vi "AddSubVIInline.vi"(9 "Numeric 3":i32, 10 "Numeric in":i32) -> (2 "Numeric out":i32)   [LabVIEW 2016]
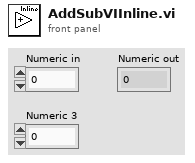
[diagram p1: front panel]
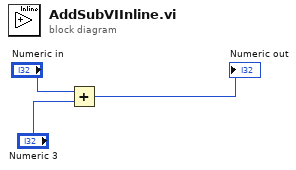
[diagram p0: block diagram]
diagram:
  n1 = Add(x="Numeric in", y="Numeric 3") -> (x+y=→"Numeric out":i32)
